vi "Stimulus trigger delay event handler.vi"   [LabVIEW 2017]
uses:
  Global Variables/FPGAstatus_Reference.vi
  User Interface/ROI Entry screen/Globals/gl_ROI Entry UI globals.vi
types:
  T1 = enum8{"Enabled", "Disabled", "Disabled and Grayed Out"}
  T2 = typedef "ROI entry screen ctrl refs cluster.ctl" = cluster{"Done button":refnum<vi>, "Imaging button":refnum<vi>, "Acquisition button":refnum<vi>, "POI dwell time (us)":refnum<vi>, "Scan dwell time per pixel (us)":refnum<vi>, "# of planes":refnum<vi>, "Zoom Ctrl":refnum<vi>, "Equal size":refnum<vi>, "Channel":refnum<vi>, "Image Display":refnum<vi>, "Z-Plane Selector":refnum<vi>, "Number of lines left":refnum<vi>, "Z-stack folder path":refnum<vi>, "POI Density":refnum<vi>, "Arb Plane Entry":refnum<vi>, "Whole plane":refnum<vi>, "Clear Last":refnum<vi>, "Clear All":refnum<vi>, "Trial Length (sec)":refnum<vi>, "Palette Type":refnum<vi>, "Intensity slider":refnum<vi>, "# POI":refnum<vi>, "Max Z Proj":refnum<vi>, "Zplane ind":refnum<vi>, "Wavelength (nm)":refnum<vi>, "Number of Trials":refnum<vi>, "Funct stim.trig.enable":refnum<vi>, "Funct stim.trig.delay (s)":refnum<vi>, "Line Mode":refnum<vi>, "Step size (µm)":refnum<vi>, "ROI move mode":refnum<vi>, "Cool-down time (s)":refnum<vi>, "Enable cool-down time":refnum<vi>, "Motor Z ind. (um)":refnum<vi>, "AOL Z ind. (um)":refnum<vi>, "Load Reference Image":refnum<vi>}
  T3 = typedef "FPGA Ref.ctl" = refnum<k20>
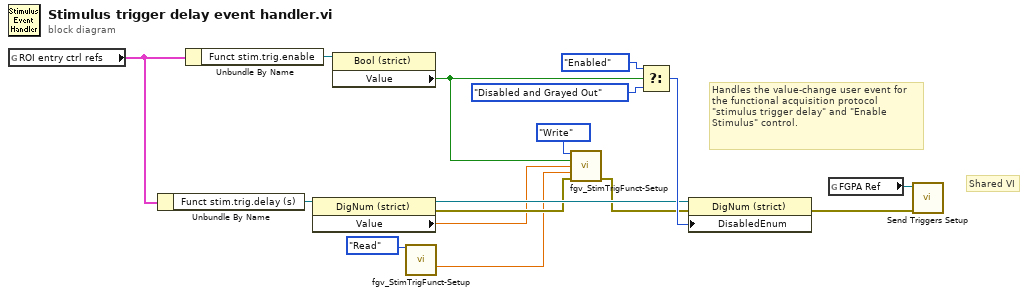
[diagram p0: block diagram]
diagram:
  # "Shared VI"
  # "Handles the value-change user event for the functional acquisition protocol \"stimulus trigger delay\" and \"Enable Stimulus\" control."
  n1 = global read "gl_ROI Entry UI globals.vi" "ROI entry ctrl refs"() -> (w9:T2)
  n2 = Unbundle By Name(w9) -> ("Funct stim.trig.delay (s)"=w14:refnum<vi>)
  n3 = Unbundle By Name(w9) -> ("Funct stim.trig.enable"=w15:refnum<vi>)
  n4 = property on="Property Node" class="DigNum (strict)"(reference=w14) -> (reference out=w7:refnum<vi>, error out=w6:errorcluster, "Value"=w2:dbl)  [unwired: 1 in]
  n5 = property on="Property Node" class="Bool (strict)"(reference=w15) -> ("Value"=w8:bool)  [unwired: 1 in, 2 out]
  n6 = call "fgv_StimTrigFunct-Setup.vi"("Function"=enum16{"Intialize", "Write", "Read", "Clear"}."Read") -> ("Funct stim.trig.width (ms)"=w1:dbl)  [unwired: 11 in, 3 out]
  n7 = call "fgv_StimTrigFunct-Setup.vi"("Function"=enum16{"Intialize", "Write", "Read", "Clear"}."Write", "Live stim.trig.enable"=w8, "Funct stim.trig.delay (sec)"=w2, "Funct stim.trig.width (ms)"=w1, "error in (no error)"=w6) -> ("error out"=w5:errorcluster)  [unwired: 7 in, 3 out]
  n8 = Select(t=T1."Enabled" ("Disabled"), s=w8, f=T1."Disabled and Grayed Out" ("Disabled")) -> (s? t:f=w12:T1)
  n9 = property on="Property Node" class="DigNum (strict)"(reference=w7, error in=w5, "DisabledEnum"=w12) -> (error out=w4:errorcluster)  [unwired: 1 out]
  n10 = global read "FPGAstatus_Reference.vi" "FGPA Ref"() -> (w16:T3)
  n11 = call "Send Triggers Setup.vi"("error in (no error)"=w4, "FGPA Ref"=w16) -> ()  [unwired: 8 in, 2 out]
